vi "PostCopyScripting.vi"(10 "MetaDataObj":refnum<class "MetaDataObj.lvclass">, 11 "User Project":refnum<vi>) -> ()   [LabVIEW 2013, in "FixedChannelTBModuleDecideFeatures.lvclass"]
uses:
  FixedChannelTBModuleDecideFeatures.lvclass
  <resource>/dialog/NewProjectWizard/MetaDataObj/MetaDataObj.lvclass
  FixedChannelTBModuleDecideFeatures.lvclass/FixedChannelTBModuleDecideFeatures.ctl
  Read component name.vi
  Read Channel Specification.vi
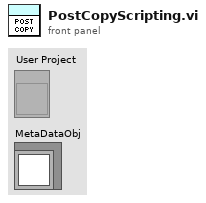
[diagram p1: front panel]
types:
  T1 = typedef "channel configuration.ctl" = cluster{"Name":string, "channel classification":T2, "data type":T3}
  T2 = typedef "TBM channel.lvclass/channel classification.ctl" = enum16{"input data", "output data", "processing parameter", "processing result"}
  T3 = typedef "tag bus.lvlib/tag descriptor.lvclass/Data Type.ctl" = enum16{"Double", "Single", "I64", "I32", "I16", "I8", "U64", "U32", "U16", "U8", "Boolean", "String", "Array of Double", "Array of Single", "Array of I64", "Array of I32", "Array of I16", "Array of I8", "Array of U64", "Array of U32", "Array of U16", "Array of U8", "Array of Boolean", "Array of String"}
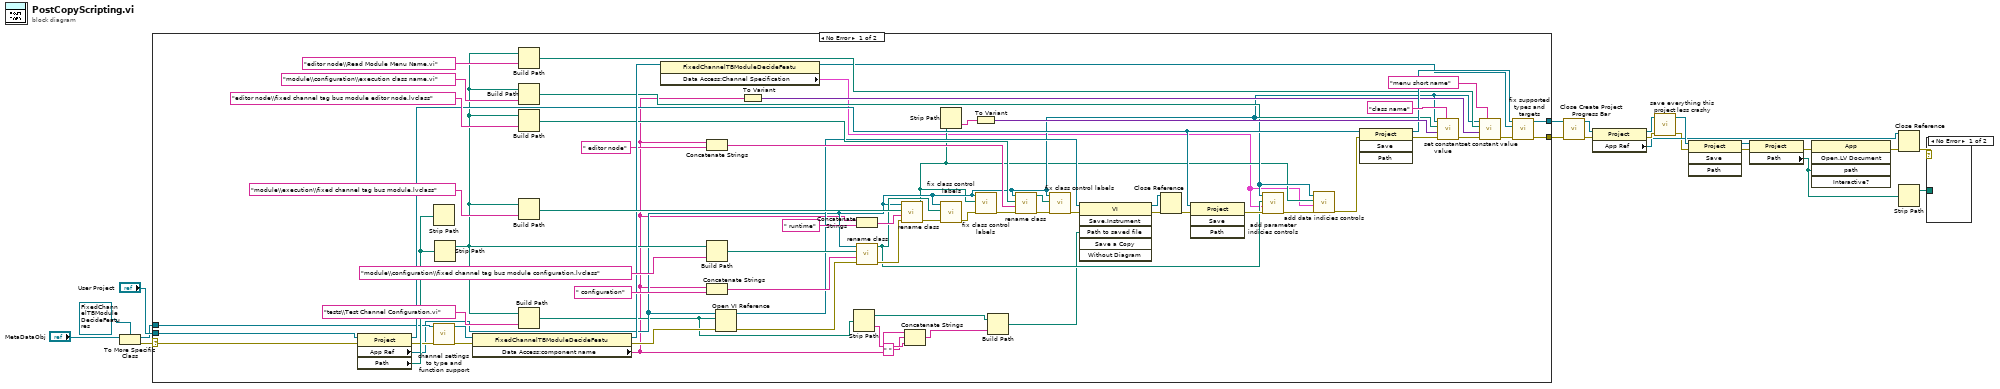
[diagram p0: block diagram]
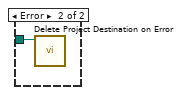
[diagram p2: hidden frame]
diagram:
  n1 = To More Specific Class(target class=refnum<class "FixedChannelTBModuleDecideFeatures.lvclass"> refnum ("DecideProjectFeatures.lvclass"), reference="MetaDataObj") -> (specific class reference=w12:refnum<class "FixedChannelTBModuleDecideFeatures.lvclass">, error out=w19:errorcluster)  [unwired: 1 in]
  n2 = case shown="No Error" w19 {
    selector: w19 -> [w44 w88]
    tunnel: [w67 w89] -> w1
    tunnel: "User Project" -> [w43 w89]
    tunnel: [w68 w88] -> w4
    tunnel: w12 -> [w46 _]
    frame No Error {
      n3 = property class="Project"(reference=w43, error in=w44) -> (reference out=w52:refnum<vi>, error out=w45:errorcluster, "App Ref"=w32:refnum<vi>, "Path"=w51:path)
      n4 = Strip Path(path=w51) -> ()  [unwired: 2 out]
      n5 = call "channel settings to type and function support.vi"("error in"=w45, "FixedChannelTBModuleDecideFeatures in"=w46) -> ("error out"=w48:errorcluster, "FixedChannelTBModuleDecideFeatures out"=w47:refnum<class "FixedChannelTBModuleDecideFeatures.lvclass">)  [unwired: 8 in]
      n6 = Strip Path(path=w51) -> (stripped path=w40:path)  [unwired: 1 out]
      n7 = property class="FixedChannelTBModuleDecideFeatu"(reference=w47, error in=w48) -> (reference out=w83:refnum<class "FixedChannelTBModuleDecideFeatures.lvclass">, error out=w49:errorcluster, "Data Access:component name"=w22:string)
      n8 = Build Path(base path=w40, name or relative path="editor node\\Read Module Menu Name.vi") -> (appended path=w59:path)
      n9 = Build Path(base path=w40, name or relative path="module\\configuration\\execution class name.vi") -> (appended path=w42:path)
      n10 = Build Path(base path=w40, name or relative path="editor node\\fixed channel tag bus module editor node.lvclass") -> (appended path=w74:path)
      n11 = Build Path(base path=w40, name or relative path="module\\execution\\fixed channel tag bus module.lvclass") -> (appended path=w85:path)
      n12 = Build Path(base path=w40, name or relative path="tests\\Test Channel Configuration.vi") -> (appended path=w28:path)
      n13 = property class="FixedChannelTBModuleDecideFeatu"(reference=w83) -> (reference out=w54:refnum<class "FixedChannelTBModuleDecideFeatures.lvclass">, "Data Access:Channel Specification"=w29:T1[])  [unwired: 1 in, 1 out]
      n14 = Concatenate Strings(w22, " editor node" ("string")) -> (w69:string)
      n15 = Build Path(base path=w40, name or relative path="module\\configuration\\fixed channel tag bus module configuration.lvclass") -> (appended path=w55:path)
      n16 = Concatenate Strings(w22, " configuration" ("string")) -> (w65:string)
      n17 = Open VI Reference(application reference (local)=w32, vi path=w28, error in (no error)=w49) -> (vi reference=w35:refnum<vi>, error out=w39:errorcluster)  [unwired: 3 in]
      n18 = To Variant(anything=w22) -> (Variant=w61:variant)
      n19 = Strip Path(path=w28) -> (stripped path=w23:path, name=w27:string)
      n20 = Concatenate Strings(w22, " runtime" ("string")) -> (w57:string)
      n21 = call "rename class.vi"("error in"=w39, "new name"=w65, "class path"=w55, "Application in"=w32) -> ("error out"=w56:errorcluster, "New Library Path"=w34:path)  [unwired: 6 in]
      n22 = call "rename class.vi"("error in"=w56, "new name"=w57, "class path"=w85, "Application in"=w32) -> ("error out"=w77:errorcluster, "New Library Path"=w30:path)  [unwired: 6 in]
      n23 = Concatenate Strings(w22, " " ("string"), w27) -> (w25:string)
      n24 = Strip Path(path=w30) -> (name=w64:string)  [unwired: 1 out]
      n25 = call "fix class control labels.vi"("error in"=w77, "class to load"=w34, "Application in"=w32) -> ("error out"=w76:errorcluster)  [unwired: 8 in]
      n26 = To Variant(anything=w64) -> (Variant=w82:variant)
      n27 = call "fix class control labels.vi"("error in"=w76, "class to load"=w30, "Application in"=w32) -> ("error out"=w71:errorcluster)  [unwired: 8 in]
      n28 = Build Path(base path=w23, name or relative path=w25) -> (appended path=w24:path)
      n29 = call "rename class.vi"("error in"=w71, "new name"=w69, "class path"=w74, "Application in"=w32) -> ("error out"=w72:errorcluster, "New Library Path"=w73:path)  [unwired: 6 in]
      n30 = call "fix class control labels.vi"("error in"=w72, "class to load"=w73, "Application in"=w32) -> ("error out"=w50:errorcluster)  [unwired: 8 in]
      n31 = invoke class="VI" method="Save.Instrument"(reference=w35, error in=w50, "Path to saved file"=w24) -> (reference out=w36:refnum<vi>, error out=w38:errorcluster)  [unwired: 3 in, 4 out]
      n32 = Close Reference(reference=w36, error in (no error)=w38) -> (error out=w37:errorcluster)
      n33 = invoke class="Project" method="Save"(reference=w52, error in=w37) -> (error out=w53:errorcluster)  [unwired: 2 in, 3 out]
      n34 = call "add parameter indicies controls.vi"("error in"=w53, "Channels to create"=w29, "cfg class path"=w34, "Application in"=w32) -> ("error out"=w33:errorcluster)  [unwired: 7 in]
      n35 = call "add data indicies controls.vi"("error in"=w33, "Channels to create"=w29, "runtime class path"=w30, "Application in"=w32) -> ("error out"=w31:errorcluster)  [unwired: 7 in]
      n36 = invoke class="Project" method="Save"(reference=w52, error in=w31) -> (reference out=w78:refnum<vi>, error out=w79:errorcluster)  [unwired: 2 in, 2 out]
      n37 = call "set constant value.vi"("control name"="class name", "error in"=w79, "data to set"=w82, "vi path"=w42, "Application in"=w32) -> ("error out"=w66:errorcluster)  [unwired: 6 in]
      n38 = call "set constant value.vi"("control name"="menu short name", "error in"=w66, "data to set"=w61, "vi path"=w59, "Application in"=w32) -> ("error out"=w63:errorcluster)  [unwired: 6 in]
      n39 = call "fix supported types and targets.vi"("error in"=w63, "DecideProjectFeatures in"=w54, "User Project in"=w78) -> ("error out"=w68:errorcluster, "User Project out"=w67:refnum<vi>)  [unwired: 7 in]
    }
    frame Error {
    }
  }
  n40 = call <resource>:"Close Create Project Progress Bar.vi"("error in (no error)"=w4, "Project"=w1) -> ("error out"=w3:errorcluster, "dup Project"=w2:refnum<vi>)  [unwired: 8 in]
  n41 = property class="Project"(reference=w2, error in=w3) -> (reference out=w9:refnum<vi>, error out=w10:errorcluster, "App Ref"=w8:refnum<vi>)
  n42 = call "save everything this project less crashy.vi"("error in"=w10, "Project in"=w9) -> ("error out"=w5:errorcluster, "Project out"=w11:refnum<vi>)  [unwired: 8 in]
  n43 = invoke class="Project" method="Save"(reference=w11, error in=w5) -> (reference out=w15:refnum<vi>, error out=w16:errorcluster)  [unwired: 2 in, 2 out]
  n44 = property class="Project"(reference=w15, error in=w16) -> (error out=w18:errorcluster, "Path"=w13:path)  [unwired: 1 out]
  n45 = invoke class="App" method="Open.LV Document"(error in=w18, "path"=w13) -> (error out=w17:errorcluster)  [unwired: 3 in, 4 out]
  n46 = Close Reference(reference=w8, error in (no error)=w17) -> (error out=w7:errorcluster)
  n47 = Strip Path(path=w13) -> (stripped path=w6:path)  [unwired: 1 out]
  n48 = case shown="No Error" w7 {
    tunnel: w6 -> [_ w90]
    frame No Error {
    }
    frame Error {
      n49 = call <resource>:"Delete Project Destination on Error.vi"("Project Destination Root"=w90) -> ()  [unwired: 11 in]
    }
  }
